vi "Test_Spectro_HR2000+.vi"() -> ()   [LabVIEW 2024]
panel:
  out "Spectrometer Name":string
  out "Number of Spectrometers":i32
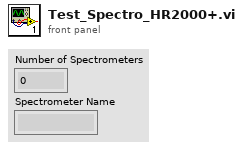
[diagram p1: front panel]
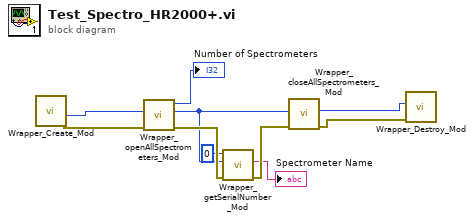
[diagram p0: block diagram]
diagram:
  n1 = call "Wrapper_Create_Mod.vi"() -> ("error out"=w8:errorcluster, "Wrapper"=w6:u32)  [unwired: 10 in]
  n2 = call "Wrapper_openAllSpectrometers_Mod.vi"("error in (no error)"=w8, "Wrapper In"=w6) -> ("error out"=w5:errorcluster, "Wrapper Out"=w2:u32, "Number of Spectrometers"=→"Number of Spectrometers":i32)  [unwired: 7 in]
  n3 = call "Wrapper_getSerialNumber_Mod.vi"("error in (no error)"=w5, "Wrapper"=w2, "Index"=0) -> ("error out"=w4:errorcluster, "Serial Number"=→"Spectrometer Name":string)  [unwired: 7 in]
  n4 = call "Wrapper_closeAllSpectrometers_Mod.vi"("error in (no error)"=w4, "Wrapper In"=w2) -> ("error out"=w10:errorcluster, "Wrapper Out"=w9:u32)  [unwired: 8 in]
  n5 = call "Wrapper_Destroy_Mod.vi"("error in (no error)"=w10, "Wrapper"=w9) -> ()  [unwired: 9 in, 1 out]
